vi "create_axis_vector_file.vi"(0 "Save folder":string, 5 "Dateiname":string, 7 "Start":dbl, 9 "Schrittlänge":dbl, 11 "# Schritte":u32) -> ()   [LabVIEW 2009]
uses:
  <vilib>/Utility/file.llb/Write To Spreadsheet File (DBL).vi
panel:
  out "Vektor":dbl[](array[numeric])
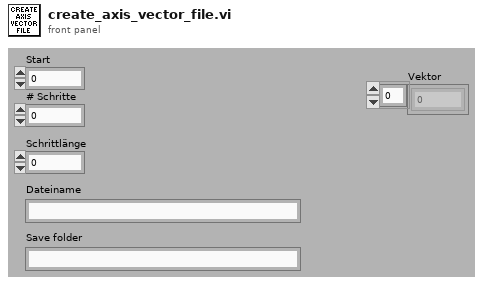
[diagram p1: front panel]
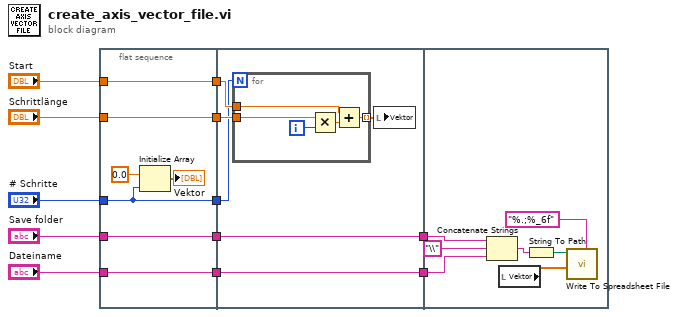
[diagram p0: block diagram]
diagram:
  n1 = flat-sequence {
    tunnel: "Save folder" -> [w16]
    tunnel: "Dateiname" -> [w17]
    tunnel: "# Schritte" -> [w13]
    tunnel: "Start" -> [w18]
    tunnel: "Schrittlänge" -> [w19]
    tunnel: [w19] -> w5
    tunnel: [w18] -> w4
    tunnel: [w13] -> w3
    tunnel: [w17] -> w2
    tunnel: [w16] -> w1
    tunnel: [w23] -> w9
    tunnel: [w22] -> w6
    tunnel: w5 -> [w25]
    tunnel: w4 -> [w24]
    tunnel: w3 -> [w20]
    tunnel: w2 -> [w23]
    tunnel: w1 -> [w22]
    tunnel: w9 -> [w33]
    tunnel: w6 -> [w32]
    frame #0 {
      n2 = Initialize Array(0.0 ("Element"), w13) -> (→"Vektor":dbl[])
    }
    frame #1 {
      n3 = for {
        N: w20 -> [_]
        tunnel: w25 -> [w29]
        tunnel: w24 -> [w27]
        tunnel: [w26] -> w21 mode=indexing
        i -> [w30]
        n4 = Multiply(x=w29, y=w30) -> (x*y=w28:dbl)
        n5 = Add(x=w27, y=w28) -> (x+y=w26:dbl)
      }
      n6 = local write "Vektor"(w21) -> ()
    }
    frame #2 {
      n7 = Concatenate Strings(w32, "\\" ("String"), w33) -> (w34:string)
      n8 = local read "Vektor"() -> (w31:dbl[])
      n9 = String To Path(string=w34) -> (path=w35:path)
      n10 = call-poly <vilib>:"Write To Spreadsheet File.vi"("format (%.3f)"="%.;%_6f", "1D data"=w31, "file path (dialog if empty)"=w35) -> ()  [unwired: 5 in, 1 out]
    }
  }
